vi "SS process.vi"(6 "AC sync source":T2, 7 "Common properties":T4={"Measurement status ref"=refnum, "TWM Status ref"=refnum, "Abort ref"=refnum, "Skip waiting ref"=refnum, "GNU Octave path"=path "C:/Program Files/GNU Octave/Octave-6.2.0/mingw64/bin", "TWM+QWTB path"=path "C:/Users/labina/Desktop/TWM-1.8.7.0-full/octprog", "lvlib path"=path "D:/martin/WAC/WACsw - github/control_software/Filter function meter/external libraries/GOLPI 0.7.3.1 source distribution LV 20.0 32 bit/lv_proc.dll", "TWM pipe"="\\\\.\\pipe\\TWM:server", "PJVS status ref"=refnum, "WAC path"=path ""}, 9 "PJVS":T5={"PJVS type"=enum."AC-supraVOLTcontrol", "Status Refnum"=refnum, "AC-supraVOLTcontrol"={"IP address:port (0.0.0.0:0000)"="0.0.0.0:0000", "Timeouts"={"TCP Read & Write (ms)"=7000, "Sensors readout"=5000, "PJVS setup"=10000, "Nullmeter readout"=5000, "Multiplexer setup"=3000, "57XX setup"=15000, "Generator setup"=5000, "Synthesizer setup"=3000, "Sampler readout"=10000}, "Simulation mode"=FALSE, "Debug mode"=FALSE}, "NPL bias source"={"DataSocketCluster"={"Server Machine"="CZC105BD8M", "Client Machine"="localhost", "Data"="P2", "TimeStamp"=0.0, "Count"=1, "Target Process"="General Server"}}, "Manual PJVS"={"PJVS frequency (Hz)"=0.0, "Reference voltages (V)"=[], "File with PJVS voltages"=path ""}, "VTT PJVS"={"some VTT only property"=""}} {"NPL bias source"."DataSocketCluster"."TimeStamp" format="%.2f"}, 10 "AC Source":T2, 11 "SS measurement":T9={"Signal frequencies (Hz)"=[1000.0], "Signal amplitudes (V)"=[0.707], "Sampling frequencies (Hz)"=[10000000.0], "Record lengths (multiples of periods)"=[10000.0], "Calculate results"=FALSE, "Algorithm"="TWM-PJVSSubS", "TWM data directories"=[], "TWM data directories relative"=[], "Settle down after AC source change (s)"=1.0, "PJVS frequencies (Hz)"=[1000.0], "PJVS reference voltages array of vector cluster"=[{"PJVS reference voltages vector"=[]}], "Requested PJVS steps"=[20], "Measure CE"=FALSE, "Measure CE before"=FALSE, "Measure CE after"=FALSE, "Single point CE measurement"=FALSE, "original CE template path"=path "", "new CE template path before SS"=path "", "new CE template path before SS relative"=path "", "new CE template path after SS"=path "", "new CE template path after SS relative"=path "", "original CE fit path"=path "", "new CE fit path before SS"=path "", "new CE fit path before SS relative"=path "", "new CE fit path after SS"=path "", "new CE fit path after SS relative"=path "", "Measure digitizer gain"=FALSE, "Measure digitizer gain before"=FALSE, "Measure digitizer gain after"=FALSE, "Digitizer gain"=0.0, "Data folder"=path "", "FR fit path"=path "", "new FR fit path relative"=path "", "Rs"=0, "Re"=0, "SS measurement info files"=[]} {"PJVS reference voltages array of vector cluster"."PJVS reference voltages vector" format="%#_3p"; "PJVS frequencies (Hz)" format="%#_3p"; "Record lengths (multiples of periods)" format="%#_3p"; "Sampling frequencies (Hz)" format="%#_3p"; "Signal amplitudes (V)" format="%#_3p"; "Signal frequencies (Hz)" format="%#_3p"}) -> (0 "error out":errorcluster)   [LabVIEW 2020]
doc: "Main VI to run whole sub sampling process. Setup devices, copy templates, calls CE measurement, SS measurement, calculation of results"
uses:
  Type definitions/SS measurement.ctl
  General AC source/Type definitions/AC Source.ctl
  General AC source/Type definitions/AC Source type.ctl
  General PJVS driver/Type definitions/PJVS.ctl
  General PJVS driver/Type definitions/PJVS Type.ctl
  external libraries/acsvcontrol-driver/Public/Type Definitions/Timeouts.ctl
  external libraries/JV modified NPL Bias source/DataSocketCluster external.ctl
  Utilities/Type definitions/Common properties.ctl
  CE Measurement/Type definitions/CE measurement.ctl
  <vilib>/Utility/error.llb/DialogType.ctl
  d155be9c-030b-4d3b-a4f2-12128ba97fa7.vi
  1648928e-eeb5-44a5-beb2-ed042b0f432d.vi
  external libraries/acsvcontrol-driver/ACSVcontrol-driver.lvlib
panel:
  out "CE measurement after":T1={"Signal frequencies (Hz) T"=[1000.0], "Signal amplitudes (V) T"=[0.707], "Sampling frequencies (Hz) T"=[10000000.0], "Record lengths (multiples of periods) T"=[10000.0], "TWM data root directory"=path "", "TWM mreasurements directories"=[], "Calculate RMS from samples"=FALSE, "Algorithm to use"="TWM-WFFT", "Quantity to read"="TWM-WFFT", "Settle down after AC source change (s) T"=1.0, "Skip PJVS setup"=FALSE, "Measurement template file"=path "", "Row of START keyword T"=0, "Row of STOP keyword T"=0, "Measurement template line T"=[], "Switch position T"=[10000.0], "FR fit mat file T"=path "", "Recalculate-skip already calculated"=FALSE} {"Switch position T" format="%#_3p"; "Record lengths (multiples of periods) T" format="%#_3p"; "Sampling frequencies (Hz) T" format="%#_3p"; "Signal amplitudes (V) T" format="%#_3p"; "Signal frequencies (Hz) T" format="%#_3p"}
  out "CE measurement before":T1={"Signal frequencies (Hz) T"=[1000.0], "Signal amplitudes (V) T"=[0.707], "Sampling frequencies (Hz) T"=[10000000.0], "Record lengths (multiples of periods) T"=[10000.0], "TWM data root directory"=path "", "TWM mreasurements directories"=[], "Calculate RMS from samples"=FALSE, "Algorithm to use"="TWM-WFFT", "Quantity to read"="TWM-WFFT", "Settle down after AC source change (s) T"=1.0, "Skip PJVS setup"=FALSE, "Measurement template file"=path "", "Row of START keyword T"=0, "Row of STOP keyword T"=0, "Measurement template line T"=[], "Switch position T"=[10000.0], "FR fit mat file T"=path "", "Recalculate-skip already calculated"=FALSE} {"Switch position T" format="%#_3p"; "Record lengths (multiples of periods) T" format="%#_3p"; "Sampling frequencies (Hz) T" format="%#_3p"; "Signal amplitudes (V) T" format="%#_3p"; "Signal frequencies (Hz) T" format="%#_3p"}
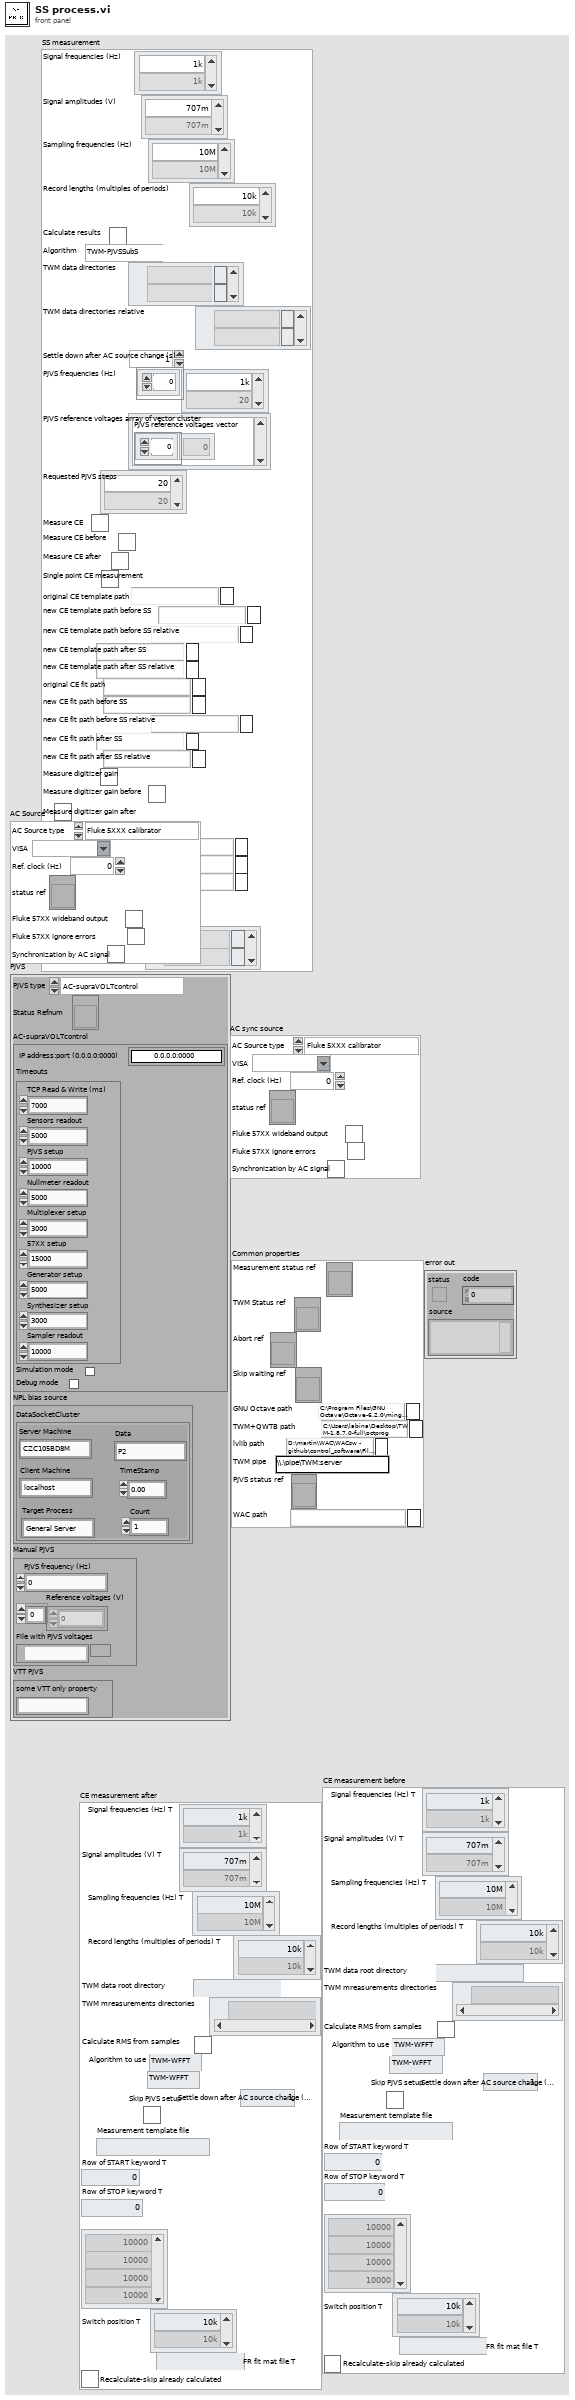
[diagram p1: front panel]
types:
  T1 = typedef "CE measurement.ctl" = cluster{"Signal frequencies (Hz) T":dbl[], "Signal amplitudes (V) T":dbl[], "Sampling frequencies (Hz) T":dbl[], "Record lengths (multiples of periods) T":dbl[], "TWM data root directory":path, "TWM mreasurements directories":path[], "Calculate RMS from samples":bool, "Algorithm to use":string, "Quantity to read":string, "Settle down after AC source change (s) T":dbl, "Skip PJVS setup":bool, "Measurement template file":path, "Row of START keyword T":i32, "Row of STOP keyword T":i32, "Measurement template line T":i32[], "Switch position T":dbl[], "FR fit mat file T":path, "Recalculate-skip already calculated":bool}
  T2 = typedef "AC Source.ctl" = cluster{"AC Source type":T3, "VISA":refnum<visa-resource-name>, "Ref. clock (Hz)":dbl, "status ref":refnum<vi>, "Fluke 57XX wideband output":bool, "Fluke 57XX ignore errors":bool, "Synchronization by AC signal":bool}
  T3 = typedef "AC Source type.ctl" = enum16{"Fluke 5XXX calibrator", "Tektronix AFG3000 series", "dummy", "Agilent 331xxA to 332xxA", "Agilent 335xxA to 336xxA"}
  T4 = typedef "Common properties.ctl" = cluster{"Measurement status ref":refnum<vi>, "TWM Status ref":refnum<vi>, "Abort ref":refnum<vi>, "Skip waiting ref":refnum<vi>, "GNU Octave path":path, "TWM+QWTB path":path, "lvlib path":path, "TWM pipe":string, "PJVS status ref":refnum<vi>, "WAC path":path}
  T5 = typedef "PJVS.ctl" = cluster{"PJVS type":T6, "Status Refnum":refnum<vi>, "AC-supraVOLTcontrol":cluster{"IP address:port (0.0.0.0:0000)":string, "Timeouts":T7, "Simulation mode":bool, "Debug mode":bool}, "NPL bias source":cluster{"DataSocketCluster":T8}, "Manual PJVS":cluster{"PJVS frequency (Hz)":dbl, "Reference voltages (V)":dbl[], "File with PJVS voltages":path}, "VTT PJVS":cluster{"some VTT only property":string}}
  T6 = typedef "PJVS Type.ctl" = enum16{"AC-supraVOLTcontrol", "JV modified NPL bias control", "Manual PJVS", "VTT PJVS"}
  T7 = typedef "ACSVcontrol-driver.lvlib/Timeouts.ctl" = cluster{"TCP Read & Write (ms)":i32, "Sensors readout":i32, "PJVS setup":i32, "Nullmeter readout":i32, "Multiplexer setup":i32, "57XX setup":i32, "Generator setup":i32, "Synthesizer setup":i32, "Sampler readout":i32}
  T8 = typedef "DataSocketCluster external.ctl" = cluster{"Server Machine":string, "Client Machine":string, "Data":string, "TimeStamp":dbl, "Count":i32, "Target Process":string}
  T9 = typedef "SS measurement.ctl" = cluster{"Signal frequencies (Hz)":dbl[], "Signal amplitudes (V)":dbl[], "Sampling frequencies (Hz)":dbl[], "Record lengths (multiples of periods)":dbl[], "Calculate results":bool, "Algorithm":string, "TWM data directories":path[], "TWM data directories relative":path[], "Settle down after AC source change (s)":dbl, "PJVS frequencies (Hz)":dbl[], "PJVS reference voltages array of vector cluster":cluster{"PJVS reference voltages vector":dbl[]}[], "Requested PJVS steps":u32[], "Measure CE":bool, "Measure CE before":bool, "Measure CE after":bool, "Single point CE measurement":bool, "original CE template path":path, "new CE template path before SS":path, "new CE template path before SS relative":path, "new CE template path after SS":path, "new CE template path after SS relative":path, "original CE fit path":path, "new CE fit path before SS":path, "new CE fit path before SS relative":path, "new CE fit path after SS":path, "new CE fit path after SS relative":path, "Measure digitizer gain":bool, "Measure digitizer gain before":bool, "Measure digitizer gain after":bool, "Digitizer gain":dbl, "Data folder":path, "FR fit path":path, "new FR fit path relative":path, "Rs":i32, "Re":i32, "SS measurement info files":path[]}
  T10 = typedef "DialogType.ctl" = u16
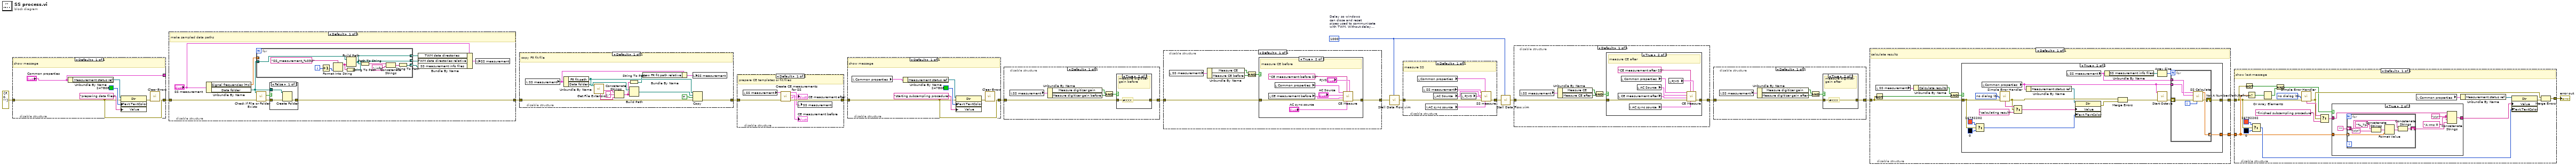
[diagram p0: block diagram]
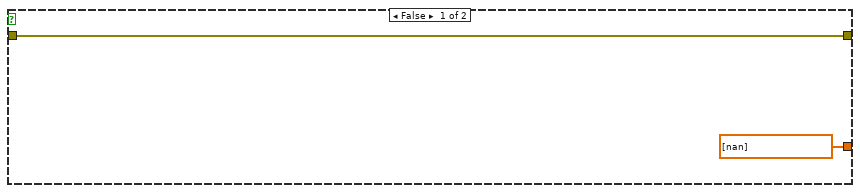
[diagram p2: hidden frame]
diagram:
  w6 = u32 1000  # Delay so windows can close and reset pipes used to communicate with TWM. Without delay error while openning pipe to TWM will appear
  n1 = disable-structure shown="Default" {
    disable-tunnel: errorcluster {"status"=FALSE, "code"=0, "source"=""} ("error constant") -> [w19]
    disable-tunnel: ["Common properties"] -> _
    disable-tunnel: [w19] -> w9
    frame Enabled {
      # "show message"
      n2 = Unbundle By Name("Common properties") -> ("Measurement status ref"=w20:refnum<vi>)
      n3 = property class="Str"(reference=w20, error in=w19, "Text.TextColor"=u32 247808 ("Text.Text Colors:Text Color"), "Value"="preparing data files") -> (error out=w22:errorcluster)  [unwired: 1 out]
      n4 = call <vilib>:"Clear Errors.vi"("error in (no error)"=w22) -> ()  [unwired: 5 in, 2 out]
    }
  }
  n5 = disable-structure shown="Default" {
    disable-tunnel: [w25] -> w13
    disable-tunnel: w9 -> [w26]
    frame Enabled {
      # "make sampled data paths"
      n6 = Unbundle By Name("SS measurement") -> ("Signal frequencies (Hz)"=w32:dbl[], "Data folder"=w24:path)
      n7 = for {
        tunnel: w24 -> [w49]
        tunnel: [w41] -> w34 mode=indexing
        tunnel: w32 -> [_] mode=indexing
        tunnel: [w44] -> w31 mode=indexing
        tunnel: [w39] -> w29 mode=indexing
        i -> [w47]
        n8 = Increment(x=w47) -> (x+1=w46:i32)
        n9 = Format Into String(format string="SS_measurement_%03d" ("string"), w46) -> (resulting string=w45:string)  [unwired: 2 in, 1 out]
        n10 = String To Path(string=w45) -> (path=w44:path)
        n11 = Build Path(base path=w49, name or relative path=w45) -> (appended path=w41:path)
        n12 = Path To String(path=w41) -> (string=w40:string)
        n13 = Concatenate Strings(w40, ".info" ("string")) -> (w43:string)
        n14 = String To Path(string=w43) -> (path=w39:path)
      }
      n15 = call <vilib>:"Check if File or Folder Exists.vi"("error in (no error)"=w26, "path"=w24) -> ("error out"=w28:errorcluster, "file or folder exists?"=w27:bool)  [unwired: 7 in, 1 out]
      n16 = case shown="False" w27 {
        tunnel: w24 -> [w37 _]
        tunnel: [w36 w38] -> w25
        tunnel: w28 -> [w35 w38]
        frame False {
          n17 = Create Folder(path (use dialog)=w37, error in=w35) -> (error out=w36:errorcluster)  [unwired: 1 in, 2 out]
        }
        frame True {
        }
      }
      n18 = Bundle By Name(cluster="SS measurement", "TWM data directories"=w34, "TWM data directories relative"=w31, "SS measurement info files"=w29) -> (w33:T9)
      n19 = local write "SS measurement"(w33) -> ()
    }
  }
  n20 = disable-structure shown="Default" {
    disable-tunnel: [w61] -> w12
    disable-tunnel: w13 -> [w62]
    frame Enabled {
      # "copy FR fit file"
      n21 = local read "SS measurement"() -> (w53:T9)
      n22 = Unbundle By Name(w53) -> ("FR fit path"=w60:path, "Data folder"=w56:path)
      n23 = call <vilib>:"Get File Extension.vi"("file"=w60) -> ("filename without extension"=w59:string, "unmodified file extension"=w57:string)  [unwired: 6 in, 3 out]
      n24 = Concatenate Strings(w59, "." ("string"), w57) -> (w52:string)
      n25 = String To Path(string=w52) -> (path=w51:path)
      n26 = Build Path(base path=w56, name or relative path=w52) -> (appended path=w55:path)
      n27 = Bundle By Name(cluster=w53, "new FR fit path relative"=w51) -> (w54:T9)
      n28 = local write "SS measurement"(w54) -> ()
      n29 = Copy(8:w62, 9:TRUE ("overwrite (F)"), 10:w55, 11:w60) -> (0:w61:errorcluster)  [unwired: 1 in, 2 out]
    }
  }
  n30 = disable-structure shown="Default" {
    disable-tunnel: w12 -> [w68]
    disable-tunnel: [w67] -> w11
    frame Enabled {
      # "prepare CE templates or fit files"
      n31 = local read "SS measurement"() -> (w66:T9)
      n32 = call "Create CE measurements for SS.vi"("error in (no error)"=w68, "SS measurement"=w66) -> ("error out"=w67:errorcluster, "CE measurement after"=→"CE measurement after":T1, "CE measurement before"=→"CE measurement before":T1, "SS measurement out"=w65:T9)  [unwired: 6 in]
      n33 = local write "SS measurement"(w65) -> ()
    }
  }
  n34 = disable-structure shown="Default" {
    disable-tunnel: w11 -> [w70]
    disable-tunnel: [w70] -> w16
    frame Enabled {
      # "show message"
      n35 = local read "Common properties"() -> (w69:T4)
      n36 = Unbundle By Name(w69) -> ("Measurement status ref"=w71:refnum<vi>)
      n37 = property class="Str"(reference=w71, error in=w70, "Text.TextColor"=u32 247808 ("Text.Text Colors:Text Color"), "Value"="starting subsampling procedure") -> (error out=w73:errorcluster)  [unwired: 1 out]
      n38 = call <vilib>:"Clear Errors.vi"("error in (no error)"=w73) -> ()  [unwired: 5 in, 2 out]
    }
  }
  n39 = disable-structure shown="Default" {
    disable-tunnel: w16 -> [w80]
    disable-tunnel: [w79] -> w14
    frame Enabled {
      n40 = local read "SS measurement"() -> (w75:T9)
      n41 = Unbundle By Name(w75) -> ("Measure digitizer gain"=w77:bool, "Measure digitizer gain before"=w78:bool)
      n42 = And(x=w77, y=w78) -> (x .and. y?=w76:bool)
      n43 = case shown="True" w76 {
        tunnel: [w81 w82] -> w79
        tunnel: w80 -> [w81 w82]
        frame False {
        }
        frame True {
          # "#XXX"
          # "measure digitizer\ngain before"
        }
      }
    }
  }
  n44 = disable-structure shown="Default" {
    disable-tunnel: [w86] -> w8
    disable-tunnel: w14 -> [w87]
    frame Enabled {
      n45 = local read "SS measurement"() -> (w88:T9)
      n46 = Unbundle By Name(w88) -> ("Measure CE"=w85:bool, "Measure CE before"=w84:bool)
      n47 = And(x=w85, y=w84) -> (x .and. y?=w83:bool)
      n48 = case shown="True" w83 {
        tunnel: w87 -> [w89 w93]
        tunnel: [w89 w92] -> w86
        frame False {
          # "only CE measurement after is planned"
        }
        frame True {
          # "measure CE before"
          n49 = local read "CE measurement before"() -> (w97:T1)
          n50 = local read "Common properties"() -> (w94:T4)
          n51 = call "CE Measure.vi"("PJVS setup"="PJVS", "AC sync source"="AC sync source", "figure prefix ()"="CE measurement before SS", "error in"=w93, "CE measurement"=w97, "AC Source"="AC Source", "Common properties"=w94) -> ("error out"=w92:errorcluster)  [unwired: 4 in]
        }
      }
    }
  }
  n52 = call "Stall Data Flow.vim"("value in"=w8, "milliseconds to wait"=w6) -> ("value out"=w7:errorcluster)  [unwired: 1 out]
  n53 = disable-structure shown="Default" {
    disable-tunnel: [w100] -> w5
    disable-tunnel: w7 -> [w101]
    frame Enabled {
      # "measure SS"
      n54 = local read "Common properties"() -> (w104:T4)
      n55 = local read "SS measurement"() -> (w102:T9)
      n56 = local read "AC sync source"() -> (w99:T2)
      n57 = local read "AC Source"() -> (w103:T2)
      n58 = local read "PJVS"() -> (w98:T5)
      n59 = call "SS measure.vi"("AC sync source"=w99, "Common properties"=w104, "error in (no error)"=w101, "PJVS"=w98, "AC Source"=w103, "SS measurement"=w102) -> ("error out"=w100:errorcluster)  [unwired: 5 in]
    }
  }
  n60 = call "Stall Data Flow.vim"("value in"=w5, "milliseconds to wait"=w6) -> ("value out"=w4:errorcluster)  [unwired: 1 out]
  n61 = disable-structure shown="Default" {
    disable-tunnel: [w106] -> w17
    disable-tunnel: w4 -> [w105]
    frame Enabled {
      n62 = local read "SS measurement"() -> (w110:T9)
      n63 = Unbundle By Name(w110) -> ("Measure CE"=w108:bool, "Measure CE after"=w107:bool)
      n64 = And(x=w108, y=w107) -> (x .and. y?=w109:bool)
      n65 = case shown="True" w109 {
        tunnel: [w111 w118] -> w106
        tunnel: w105 -> [w111 w119]
        frame False {
          # "no CE measurement after, nothing to do"
        }
        frame True {
          # "measure CE after"
          n66 = local read "CE measurement after"() -> (w113:T1)
          n67 = local read "Common properties"() -> (w114:T4)
          n68 = local read "AC sync source"() -> (w117:T2)
          n69 = local read "AC Source"() -> (w116:T2)
          n70 = local read "PJVS"() -> (w115:T5)
          n71 = call "CE Measure.vi"("PJVS setup"=w115, "AC sync source"=w117, "figure prefix ()"="CE measurement after SS", "error in"=w119, "CE measurement"=w113, "AC Source"=w116, "Common properties"=w114) -> ("error out"=w118:errorcluster)  [unwired: 4 in]
        }
      }
    }
  }
  n72 = disable-structure shown="Default" {
    disable-tunnel: w17 -> [w121]
    disable-tunnel: [w120] -> w3
    frame Enabled {
      n73 = local read "SS measurement"() -> (w125:T9)
      n74 = Unbundle By Name(w125) -> ("Measure digitizer gain"=w122:bool, "Measure digitizer gain after"=w123:bool)
      n75 = And(x=w122, y=w123) -> (x .and. y?=w124:bool)
      n76 = case shown="True" w124 {
        tunnel: [w126 w127] -> w120
        tunnel: w121 -> [w126 w127]
        frame False {
        }
        frame True {
          # "#XXX"
          # "measure digitizer\ngain after"
        }
      }
    }
  }
  n77 = disable-structure shown="Default" {
    disable-tunnel: w3 -> [w130]
    disable-tunnel: [w131] -> w2
    disable-tunnel: [w128] -> w1
    frame Enabled {
      # "calculate results"
      n78 = Not(x=w130) -> (.not. x?=w129:bool)
      n79 = local read "SS measurement"() -> (w134:T9)
      n80 = Unbundle By Name(w134) -> ("Calculate results"=w133:bool)
      n81 = And(x=w133, y=w129) -> (x .and. y?=w132:bool)
      n82 = case shown="True" w132 {
        tunnel: w130 -> [w136 w145]
        tunnel: [w136 w143] -> w131
        tunnel: [dbl[] [nan] w137] -> w128
        frame False {
        }
        frame True {
          w152 = T10 0 items=["no dialog", "OK message", "continue or stop message", "OK message + warnings", "continue/stop + warnings"] ("type of dialog (OK msg:1)")
          n83 = Select(t=u32 16732202 ("Text.Text Colors:Text Color"), s=w145, f=u32 0 ("Text.Text Colors:Text Color")) -> (s? t:f=w149:u32)
          n84 = local read "Common properties"() -> (w141:T4)
          n85 = call <vilib>:"Simple Error Handler.vi"("type of dialog (OK msg:1)"=w152, "error in (no error)"=w145) -> ("error out"=w147:errorcluster, "message"=w155:string)  [unwired: 3 in, 3 out]
          n86 = Select(t=w155, s=w147, f="calculating result") -> (s? t:f=w153:string)
          n87 = Unbundle By Name(w141) -> ("Measurement status ref"=w146:refnum<vi>)
          n88 = local read "SS measurement"() -> (w140:T9)
          n89 = property class="Str"(reference=w146, "Value"=w153, "Text.TextColor"=w149) -> (error out=w148:errorcluster)  [unwired: 1 in, 1 out]
          n90 = Unbundle By Name(w140) -> ("SS measurement info files"=w139:path[])
          n91 = Merge Errors(w147, w148) -> (w144:errorcluster)
          n92 = Array Size(array=w139) -> (size(s)=w138:i32)
          n93 = call "Start Octave.vi"("error in (no error)"=w144, "Common properties"=w141) -> ("error out"=w142:errorcluster)  [unwired: 9 in]
          n94 = for {
            N: w138 -> [_]
            tunnel: w140 -> [w159]
            tunnel: w141 -> [w158]
            shift-right: [w161] -> w143
            shift-left: w142 -> [w160]
            tunnel: [w156] -> w137 mode=indexing
            i -> [w157]
            n95 = call "SS Calculate.vi"("index"=w157, "error in (no error)"=w160, "SS measurement"=w159, "Common properties"=w158) -> ("error out"=w161:errorcluster, "value"=w156:dbl)  [unwired: 6 in]
          }
        }
      }
    }
  }
  n96 = disable-structure shown="Default" {
    disable-tunnel: [w170] -> w15
    disable-tunnel: w2 -> [w164]
    disable-tunnel: w1 -> [w168]
    frame Enabled {
      w178 = T10 0 items=["no dialog", "OK message", "continue or stop message", "OK message + warnings", "continue/stop + warnings"] ("type of dialog (OK msg:1)")
      # "show last message"
      n97 = Not(x=w164) -> (.not. x?=w165:bool)
      n98 = Not A Number/Path/Refnum?(number/path/refnum=w168) -> (NaN/Path/Refnum?=w169:bool[])
      n99 = Select(t=u32 16732202 ("Text.Text Colors:Text Color"), s=w164, f=u32 0 ("Text.Text Colors:Text Color")) -> (s? t:f=w175:u32)
      n100 = Or Array Elements(Boolean array=w169) -> (logical OR=w167:bool)
      n101 = And(x=w165, y=w167) -> (x .and. y?=w166:bool)
      n102 = call <vilib>:"Simple Error Handler.vi"("type of dialog (OK msg:1)"=w178, "error in (no error)"=w164) -> ("error out"=w173:errorcluster, "message"=w180:string)  [unwired: 3 in, 3 out]
      n103 = Select(t=w180, s=w173, f="finished subsampling procedure") -> (s? t:f=w163:string)
      n104 = case shown="True" w166 {
        tunnel: w168 -> [_ w187]
        tunnel: [w181 w184] -> w162
        tunnel: w163 -> [w181 w186]
        frame False {
        }
        frame True {
          w182 = "\r\n"
          n105 = for {
            tunnel: w187 -> [w195] mode=indexing
            shift-right: [w190] -> w185
            shift-left: "" -> [w191]
            n106 = Concatenate Strings("%_7p," ("format string"), "\r\n") -> (w192:string)
            n107 = Format Value(format string=w192, value (0)=w195) -> (output string=w189:string)  [unwired: 1 in]
            n108 = Concatenate Strings(w191, w189) -> (w190:string)
          }
          n109 = Concatenate Strings(w186, w182, "A rms = " ("string"), w182, w185) -> (w184:string)
        }
      }
      n110 = local read "Common properties"() -> (w171:T4)
      n111 = Unbundle By Name(w171) -> ("Measurement status ref"=w172:refnum<vi>)
      n112 = property class="Str"(reference=w172, "Value"=w162, "Text.TextColor"=w175) -> (error out=w174:errorcluster)  [unwired: 1 in, 1 out]
      n113 = Merge Errors(w173, w174) -> (w170:errorcluster)
    }
  }
  "error out" <- w15
